vi "Main.vi"() -> ()   [LabVIEW 2021] (continued)
                    w821 = T9 37 items=["刷新间隔", "波特率", "布尔1设置项", "布尔2设置项", "布尔3设置项", "布尔4设置项", "布尔5设置项", "布尔6设置项", "布尔7设置项", "布尔8设置项", "显控1设置", "显控2设置", "显控3设置", "显控4设置", "显控5设置", "显控6设置", "显控7设置", "显控8设置", "显控9设置", "显控10设置", "显控11设置", "显控12设置", "设控1设置", "设控2设置", "设控3设置", "设控4设置", "设控5设置", "设控6设置", "设控7设置", "设控8设置", "曲线1设置", "曲线2设置", "曲线3设置", "曲线4设置", "曲线5设置", "曲线6设置", "曲线7设置", "曲线8设置", "曲线9设置", "曲线10设置", "曲线11设置", "曲线12设置", "曲线13设置", "曲线14设置", "曲线15设置", "曲线16设置", "曲线17设置", "曲线18设置", "曲线19设置", "曲线20设置", "曲线21设置", "曲线22设置", "曲线23设置", "曲线24设置", "曲线25设置", "曲线26设置", "曲线27设置", "曲线28设置", "曲线29设置", "曲线30设置", "曲线31设置", "曲线32设置", "曲线33设置", "曲线34设置", "曲线35设置", "曲线36设置", "曲线37设置", "曲线38设置", "曲线39设置", "曲线40设置", "曲线41设置", "曲线42设置", "曲线43设置", "曲线44设置", "曲线45设置", "曲线46设置", "曲线47设置", "曲线48设置", "曲线49设置", "曲线50设置", "曲线51设置", "曲线52设置", "曲线53设置", "曲线54设置", "曲线55设置", "曲线56设置", "曲线57设置", "曲线58设置", "曲线59设置", "曲线60设置", "曲线61设置", "曲线62设置", "曲线63设置", "曲线64设置", "ID值", "数据模式"] ("DataInitDef")
                    n650 = property on="表格" class="Tbl (严格)"() -> ("Selection Start"=w831:T1)  [unwired: 2 in, 2 out]
                    n651 = Unbundle By Name(w831) -> ("Row"=w829:i32)
                    n652 = property on="表格" class="Tbl (严格)"() -> ("Value"=w830:string[][])  [unwired: 2 in, 2 out]
                    n653 = Number To Decimal String(number=w829) -> (decimal integer string=w828:string)  [unwired: 1 in]
                    n654 = Index Array(array=w830, index (row)=w829, index (col)=0 ("禁用的索引 (列)")) -> (element=w827:string)
                    n655 = String Subset(string=w827, length (rest)=16 ("长度（剩余）")) -> (substring=w826:string)  [unwired: 1 in]
                    n656 = property on="曲线8设置" class="Str"("Val(Sgnl)"=w826) -> ()  [unwired: 2 in, 2 out]
                    n657 = invoke on="控件配置文件" class="Tbl (严格)" method="Set Cell Value"("X Index"=1 ("X索引"), "Y Index"=w821, "Value"=w828) -> ()  [unwired: 3 in, 6 out]
                    n658 = invoke on="控件配置文件" class="Tbl (严格)" method="Set Cell Value"("X Index"=0 ("X索引"), "Y Index"=w821, "Value"=w826) -> ()  [unwired: 3 in, 6 out]
                  }
                  frame "关联到曲线9" {
                    w832 = T9 38 items=["刷新间隔", "波特率", "布尔1设置项", "布尔2设置项", "布尔3设置项", "布尔4设置项", "布尔5设置项", "布尔6设置项", "布尔7设置项", "布尔8设置项", "显控1设置", "显控2设置", "显控3设置", "显控4设置", "显控5设置", "显控6设置", "显控7设置", "显控8设置", "显控9设置", "显控10设置", "显控11设置", "显控12设置", "设控1设置", "设控2设置", "设控3设置", "设控4设置", "设控5设置", "设控6设置", "设控7设置", "设控8设置", "曲线1设置", "曲线2设置", "曲线3设置", "曲线4设置", "曲线5设置", "曲线6设置", "曲线7设置", "曲线8设置", "曲线9设置", "曲线10设置", "曲线11设置", "曲线12设置", "曲线13设置", "曲线14设置", "曲线15设置", "曲线16设置", "曲线17设置", "曲线18设置", "曲线19设置", "曲线20设置", "曲线21设置", "曲线22设置", "曲线23设置", "曲线24设置", "曲线25设置", "曲线26设置", "曲线27设置", "曲线28设置", "曲线29设置", "曲线30设置", "曲线31设置", "曲线32设置", "曲线33设置", "曲线34设置", "曲线35设置", "曲线36设置", "曲线37设置", "曲线38设置", "曲线39设置", "曲线40设置", "曲线41设置", "曲线42设置", "曲线43设置", "曲线44设置", "曲线45设置", "曲线46设置", "曲线47设置", "曲线48设置", "曲线49设置", "曲线50设置", "曲线51设置", "曲线52设置", "曲线53设置", "曲线54设置", "曲线55设置", "曲线56设置", "曲线57设置", "曲线58设置", "曲线59设置", "曲线60设置", "曲线61设置", "曲线62设置", "曲线63设置", "曲线64设置", "ID值", "数据模式"] ("DataInitDef")
                    n659 = property on="表格" class="Tbl (严格)"() -> ("Selection Start"=w842:T1)  [unwired: 2 in, 2 out]
                    n660 = Unbundle By Name(w842) -> ("Row"=w840:i32)
                    n661 = property on="表格" class="Tbl (严格)"() -> ("Value"=w841:string[][])  [unwired: 2 in, 2 out]
                    n662 = Number To Decimal String(number=w840) -> (decimal integer string=w839:string)  [unwired: 1 in]
                    n663 = Index Array(array=w841, index (row)=w840, index (col)=0 ("禁用的索引 (列)")) -> (element=w838:string)
                    n664 = String Subset(string=w838, length (rest)=16 ("长度（剩余）")) -> (substring=w837:string)  [unwired: 1 in]
                    n665 = property on="曲线9设置" class="Str"("Val(Sgnl)"=w837) -> ()  [unwired: 2 in, 2 out]
                    n666 = invoke on="控件配置文件" class="Tbl (严格)" method="Set Cell Value"("X Index"=1 ("X索引"), "Y Index"=w832, "Value"=w839) -> ()  [unwired: 3 in, 6 out]
                    n667 = invoke on="控件配置文件" class="Tbl (严格)" method="Set Cell Value"("X Index"=0 ("X索引"), "Y Index"=w832, "Value"=w837) -> ()  [unwired: 3 in, 6 out]
                  }
                  frame "关联到曲线10" {
                    w843 = T9 39 items=["刷新间隔", "波特率", "布尔1设置项", "布尔2设置项", "布尔3设置项", "布尔4设置项", "布尔5设置项", "布尔6设置项", "布尔7设置项", "布尔8设置项", "显控1设置", "显控2设置", "显控3设置", "显控4设置", "显控5设置", "显控6设置", "显控7设置", "显控8设置", "显控9设置", "显控10设置", "显控11设置", "显控12设置", "设控1设置", "设控2设置", "设控3设置", "设控4设置", "设控5设置", "设控6设置", "设控7设置", "设控8设置", "曲线1设置", "曲线2设置", "曲线3设置", "曲线4设置", "曲线5设置", "曲线6设置", "曲线7设置", "曲线8设置", "曲线9设置", "曲线10设置", "曲线11设置", "曲线12设置", "曲线13设置", "曲线14设置", "曲线15设置", "曲线16设置", "曲线17设置", "曲线18设置", "曲线19设置", "曲线20设置", "曲线21设置", "曲线22设置", "曲线23设置", "曲线24设置", "曲线25设置", "曲线26设置", "曲线27设置", "曲线28设置", "曲线29设置", "曲线30设置", "曲线31设置", "曲线32设置", "曲线33设置", "曲线34设置", "曲线35设置", "曲线36设置", "曲线37设置", "曲线38设置", "曲线39设置", "曲线40设置", "曲线41设置", "曲线42设置", "曲线43设置", "曲线44设置", "曲线45设置", "曲线46设置", "曲线47设置", "曲线48设置", "曲线49设置", "曲线50设置", "曲线51设置", "曲线52设置", "曲线53设置", "曲线54设置", "曲线55设置", "曲线56设置", "曲线57设置", "曲线58设置", "曲线59设置", "曲线60设置", "曲线61设置", "曲线62设置", "曲线63设置", "曲线64设置", "ID值", "数据模式"] ("DataInitDef")
                    n668 = property on="表格" class="Tbl (严格)"() -> ("Selection Start"=w848:T1)  [unwired: 2 in, 2 out]
                    n669 = Unbundle By Name(w848) -> ("Row"=w850:i32)
                    n670 = property on="表格" class="Tbl (严格)"() -> ("Value"=w849:string[][])  [unwired: 2 in, 2 out]
                    n671 = Number To Decimal String(number=w850) -> (decimal integer string=w851:string)  [unwired: 1 in]
                    n672 = Index Array(array=w849, index (row)=w850, index (col)=0 ("禁用的索引 (列)")) -> (element=w852:string)
                    n673 = String Subset(string=w852, length (rest)=16 ("长度（剩余）")) -> (substring=w853:string)  [unwired: 1 in]
                    n674 = property on="曲线10设置" class="Str"("Val(Sgnl)"=w853) -> ()  [unwired: 2 in, 2 out]
                    n675 = invoke on="控件配置文件" class="Tbl (严格)" method="Set Cell Value"("X Index"=1 ("X索引"), "Y Index"=w843, "Value"=w851) -> ()  [unwired: 3 in, 6 out]
                    n676 = invoke on="控件配置文件" class="Tbl (严格)" method="Set Cell Value"("X Index"=0 ("X索引"), "Y Index"=w843, "Value"=w853) -> ()  [unwired: 3 in, 6 out]
                  }
                  frame "关联到曲线11" {
                    w854 = T9 40 items=["刷新间隔", "波特率", "布尔1设置项", "布尔2设置项", "布尔3设置项", "布尔4设置项", "布尔5设置项", "布尔6设置项", "布尔7设置项", "布尔8设置项", "显控1设置", "显控2设置", "显控3设置", "显控4设置", "显控5设置", "显控6设置", "显控7设置", "显控8设置", "显控9设置", "显控10设置", "显控11设置", "显控12设置", "设控1设置", "设控2设置", "设控3设置", "设控4设置", "设控5设置", "设控6设置", "设控7设置", "设控8设置", "曲线1设置", "曲线2设置", "曲线3设置", "曲线4设置", "曲线5设置", "曲线6设置", "曲线7设置", "曲线8设置", "曲线9设置", "曲线10设置", "曲线11设置", "曲线12设置", "曲线13设置", "曲线14设置", "曲线15设置", "曲线16设置", "曲线17设置", "曲线18设置", "曲线19设置", "曲线20设置", "曲线21设置", "曲线22设置", "曲线23设置", "曲线24设置", "曲线25设置", "曲线26设置", "曲线27设置", "曲线28设置", "曲线29设置", "曲线30设置", "曲线31设置", "曲线32设置", "曲线33设置", "曲线34设置", "曲线35设置", "曲线36设置", "曲线37设置", "曲线38设置", "曲线39设置", "曲线40设置", "曲线41设置", "曲线42设置", "曲线43设置", "曲线44设置", "曲线45设置", "曲线46设置", "曲线47设置", "曲线48设置", "曲线49设置", "曲线50设置", "曲线51设置", "曲线52设置", "曲线53设置", "曲线54设置", "曲线55设置", "曲线56设置", "曲线57设置", "曲线58设置", "曲线59设置", "曲线60设置", "曲线61设置", "曲线62设置", "曲线63设置", "曲线64设置", "ID值", "数据模式"] ("DataInitDef")
                    n677 = property on="表格" class="Tbl (严格)"() -> ("Selection Start"=w859:T1)  [unwired: 2 in, 2 out]
                    n678 = Unbundle By Name(w859) -> ("Row"=w861:i32)
                    n679 = property on="表格" class="Tbl (严格)"() -> ("Value"=w860:string[][])  [unwired: 2 in, 2 out]
                    n680 = Number To Decimal String(number=w861) -> (decimal integer string=w862:string)  [unwired: 1 in]
                    n681 = Index Array(array=w860, index (row)=w861, index (col)=0 ("禁用的索引 (列)")) -> (element=w863:string)
                    n682 = String Subset(string=w863, length (rest)=16 ("长度（剩余）")) -> (substring=w864:string)  [unwired: 1 in]
                    n683 = property on="曲线11设置" class="Str"("Val(Sgnl)"=w864) -> ()  [unwired: 2 in, 2 out]
                    n684 = invoke on="控件配置文件" class="Tbl (严格)" method="Set Cell Value"("X Index"=1 ("X索引"), "Y Index"=w854, "Value"=w862) -> ()  [unwired: 3 in, 6 out]
                    n685 = invoke on="控件配置文件" class="Tbl (严格)" method="Set Cell Value"("X Index"=0 ("X索引"), "Y Index"=w854, "Value"=w864) -> ()  [unwired: 3 in, 6 out]
                  }
                  frame "关联到曲线12" {
                    w865 = T9 41 items=["刷新间隔", "波特率", "布尔1设置项", "布尔2设置项", "布尔3设置项", "布尔4设置项", "布尔5设置项", "布尔6设置项", "布尔7设置项", "布尔8设置项", "显控1设置", "显控2设置", "显控3设置", "显控4设置", "显控5设置", "显控6设置", "显控7设置", "显控8设置", "显控9设置", "显控10设置", "显控11设置", "显控12设置", "设控1设置", "设控2设置", "设控3设置", "设控4设置", "设控5设置", "设控6设置", "设控7设置", "设控8设置", "曲线1设置", "曲线2设置", "曲线3设置", "曲线4设置", "曲线5设置", "曲线6设置", "曲线7设置", "曲线8设置", "曲线9设置", "曲线10设置", "曲线11设置", "曲线12设置", "曲线13设置", "曲线14设置", "曲线15设置", "曲线16设置", "曲线17设置", "曲线18设置", "曲线19设置", "曲线20设置", "曲线21设置", "曲线22设置", "曲线23设置", "曲线24设置", "曲线25设置", "曲线26设置", "曲线27设置", "曲线28设置", "曲线29设置", "曲线30设置", "曲线31设置", "曲线32设置", "曲线33设置", "曲线34设置", "曲线35设置", "曲线36设置", "曲线37设置", "曲线38设置", "曲线39设置", "曲线40设置", "曲线41设置", "曲线42设置", "曲线43设置", "曲线44设置", "曲线45设置", "曲线46设置", "曲线47设置", "曲线48设置", "曲线49设置", "曲线50设置", "曲线51设置", "曲线52设置", "曲线53设置", "曲线54设置", "曲线55设置", "曲线56设置", "曲线57设置", "曲线58设置", "曲线59设置", "曲线60设置", "曲线61设置", "曲线62设置", "曲线63设置", "曲线64设置", "ID值", "数据模式"] ("DataInitDef")
                    n686 = property on="表格" class="Tbl (严格)"() -> ("Selection Start"=w870:T1)  [unwired: 2 in, 2 out]
                    n687 = Unbundle By Name(w870) -> ("Row"=w872:i32)
                    n688 = property on="表格" class="Tbl (严格)"() -> ("Value"=w871:string[][])  [unwired: 2 in, 2 out]
                    n689 = Number To Decimal String(number=w872) -> (decimal integer string=w873:string)  [unwired: 1 in]
                    n690 = Index Array(array=w871, index (row)=w872, index (col)=0 ("禁用的索引 (列)")) -> (element=w874:string)
                    n691 = String Subset(string=w874, length (rest)=16 ("长度（剩余）")) -> (substring=w875:string)  [unwired: 1 in]
                    n692 = property on="曲线12设置" class="Str"("Val(Sgnl)"=w875) -> ()  [unwired: 2 in, 2 out]
                    n693 = invoke on="控件配置文件" class="Tbl (严格)" method="Set Cell Value"("X Index"=1 ("X索引"), "Y Index"=w865, "Value"=w873) -> ()  [unwired: 3 in, 6 out]
                    n694 = invoke on="控件配置文件" class="Tbl (严格)" method="Set Cell Value"("X Index"=0 ("X索引"), "Y Index"=w865, "Value"=w875) -> ()  [unwired: 3 in, 6 out]
                  }
                  frame "关联到曲线13" {
                    w876 = T9 42 items=["刷新间隔", "波特率", "布尔1设置项", "布尔2设置项", "布尔3设置项", "布尔4设置项", "布尔5设置项", "布尔6设置项", "布尔7设置项", "布尔8设置项", "显控1设置", "显控2设置", "显控3设置", "显控4设置", "显控5设置", "显控6设置", "显控7设置", "显控8设置", "显控9设置", "显控10设置", "显控11设置", "显控12设置", "设控1设置", "设控2设置", "设控3设置", "设控4设置", "设控5设置", "设控6设置", "设控7设置", "设控8设置", "曲线1设置", "曲线2设置", "曲线3设置", "曲线4设置", "曲线5设置", "曲线6设置", "曲线7设置", "曲线8设置", "曲线9设置", "曲线10设置", "曲线11设置", "曲线12设置", "曲线13设置", "曲线14设置", "曲线15设置", "曲线16设置", "曲线17设置", "曲线18设置", "曲线19设置", "曲线20设置", "曲线21设置", "曲线22设置", "曲线23设置", "曲线24设置", "曲线25设置", "曲线26设置", "曲线27设置", "曲线28设置", "曲线29设置", "曲线30设置", "曲线31设置", "曲线32设置", "曲线33设置", "曲线34设置", "曲线35设置", "曲线36设置", "曲线37设置", "曲线38设置", "曲线39设置", "曲线40设置", "曲线41设置", "曲线42设置", "曲线43设置", "曲线44设置", "曲线45设置", "曲线46设置", "曲线47设置", "曲线48设置", "曲线49设置", "曲线50设置", "曲线51设置", "曲线52设置", "曲线53设置", "曲线54设置", "曲线55设置", "曲线56设置", "曲线57设置", "曲线58设置", "曲线59设置", "曲线60设置", "曲线61设置", "曲线62设置", "曲线63设置", "曲线64设置", "ID值", "数据模式"] ("DataInitDef")
                    n695 = property on="表格" class="Tbl (严格)"() -> ("Selection Start"=w881:T1)  [unwired: 2 in, 2 out]
                    n696 = Unbundle By Name(w881) -> ("Row"=w883:i32)
                    n697 = property on="表格" class="Tbl (严格)"() -> ("Value"=w882:string[][])  [unwired: 2 in, 2 out]
                    n698 = Number To Decimal String(number=w883) -> (decimal integer string=w884:string)  [unwired: 1 in]
                    n699 = Index Array(array=w882, index (row)=w883, index (col)=0 ("禁用的索引 (列)")) -> (element=w885:string)
                    n700 = String Subset(string=w885, length (rest)=16 ("长度（剩余）")) -> (substring=w886:string)  [unwired: 1 in]
                    n701 = property on="曲线13设置" class="Str"("Val(Sgnl)"=w886) -> ()  [unwired: 2 in, 2 out]
                    n702 = invoke on="控件配置文件" class="Tbl (严格)" method="Set Cell Value"("X Index"=1 ("X索引"), "Y Index"=w876, "Value"=w884) -> ()  [unwired: 3 in, 6 out]
                    n703 = invoke on="控件配置文件" class="Tbl (严格)" method="Set Cell Value"("X Index"=0 ("X索引"), "Y Index"=w876, "Value"=w886) -> ()  [unwired: 3 in, 6 out]
                  }
                  frame "关联到曲线14" {
                    w887 = T9 43 items=["刷新间隔", "波特率", "布尔1设置项", "布尔2设置项", "布尔3设置项", "布尔4设置项", "布尔5设置项", "布尔6设置项", "布尔7设置项", "布尔8设置项", "显控1设置", "显控2设置", "显控3设置", "显控4设置", "显控5设置", "显控6设置", "显控7设置", "显控8设置", "显控9设置", "显控10设置", "显控11设置", "显控12设置", "设控1设置", "设控2设置", "设控3设置", "设控4设置", "设控5设置", "设控6设置", "设控7设置", "设控8设置", "曲线1设置", "曲线2设置", "曲线3设置", "曲线4设置", "曲线5设置", "曲线6设置", "曲线7设置", "曲线8设置", "曲线9设置", "曲线10设置", "曲线11设置", "曲线12设置", "曲线13设置", "曲线14设置", "曲线15设置", "曲线16设置", "曲线17设置", "曲线18设置", "曲线19设置", "曲线20设置", "曲线21设置", "曲线22设置", "曲线23设置", "曲线24设置", "曲线25设置", "曲线26设置", "曲线27设置", "曲线28设置", "曲线29设置", "曲线30设置", "曲线31设置", "曲线32设置", "曲线33设置", "曲线34设置", "曲线35设置", "曲线36设置", "曲线37设置", "曲线38设置", "曲线39设置", "曲线40设置", "曲线41设置", "曲线42设置", "曲线43设置", "曲线44设置", "曲线45设置", "曲线46设置", "曲线47设置", "曲线48设置", "曲线49设置", "曲线50设置", "曲线51设置", "曲线52设置", "曲线53设置", "曲线54设置", "曲线55设置", "曲线56设置", "曲线57设置", "曲线58设置", "曲线59设置", "曲线60设置", "曲线61设置", "曲线62设置", "曲线63设置", "曲线64设置", "ID值", "数据模式"] ("DataInitDef")
                    n704 = property on="表格" class="Tbl (严格)"() -> ("Selection Start"=w892:T1)  [unwired: 2 in, 2 out]
                    n705 = Unbundle By Name(w892) -> ("Row"=w894:i32)
                    n706 = property on="表格" class="Tbl (严格)"() -> ("Value"=w893:string[][])  [unwired: 2 in, 2 out]
                    n707 = Number To Decimal String(number=w894) -> (decimal integer string=w895:string)  [unwired: 1 in]
                    n708 = Index Array(array=w893, index (row)=w894, index (col)=0 ("禁用的索引 (列)")) -> (element=w896:string)
                    n709 = String Subset(string=w896, length (rest)=16 ("长度（剩余）")) -> (substring=w897:string)  [unwired: 1 in]
                    n710 = property on="曲线14设置" class="Str"("Val(Sgnl)"=w897) -> ()  [unwired: 2 in, 2 out]
                    n711 = invoke on="控件配置文件" class="Tbl (严格)" method="Set Cell Value"("X Index"=1 ("X索引"), "Y Index"=w887, "Value"=w895) -> ()  [unwired: 3 in, 6 out]
                    n712 = invoke on="控件配置文件" class="Tbl (严格)" method="Set Cell Value"("X Index"=0 ("X索引"), "Y Index"=w887, "Value"=w897) -> ()  [unwired: 3 in, 6 out]
                  }
                  frame "关联到曲线15" {
                    w898 = T9 44 items=["刷新间隔", "波特率", "布尔1设置项", "布尔2设置项", "布尔3设置项", "布尔4设置项", "布尔5设置项", "布尔6设置项", "布尔7设置项", "布尔8设置项", "显控1设置", "显控2设置", "显控3设置", "显控4设置", "显控5设置", "显控6设置", "显控7设置", "显控8设置", "显控9设置", "显控10设置", "显控11设置", "显控12设置", "设控1设置", "设控2设置", "设控3设置", "设控4设置", "设控5设置", "设控6设置", "设控7设置", "设控8设置", "曲线1设置", "曲线2设置", "曲线3设置", "曲线4设置", "曲线5设置", "曲线6设置", "曲线7设置", "曲线8设置", "曲线9设置", "曲线10设置", "曲线11设置", "曲线12设置", "曲线13设置", "曲线14设置", "曲线15设置", "曲线16设置", "曲线17设置", "曲线18设置", "曲线19设置", "曲线20设置", "曲线21设置", "曲线22设置", "曲线23设置", "曲线24设置", "曲线25设置", "曲线26设置", "曲线27设置", "曲线28设置", "曲线29设置", "曲线30设置", "曲线31设置", "曲线32设置", "曲线33设置", "曲线34设置", "曲线35设置", "曲线36设置", "曲线37设置", "曲线38设置", "曲线39设置", "曲线40设置", "曲线41设置", "曲线42设置", "曲线43设置", "曲线44设置", "曲线45设置", "曲线46设置", "曲线47设置", "曲线48设置", "曲线49设置", "曲线50设置", "曲线51设置", "曲线52设置", "曲线53设置", "曲线54设置", "曲线55设置", "曲线56设置", "曲线57设置", "曲线58设置", "曲线59设置", "曲线60设置", "曲线61设置", "曲线62设置", "曲线63设置", "曲线64设置", "ID值", "数据模式"] ("DataInitDef")
                    n713 = property on="表格" class="Tbl (严格)"() -> ("Selection Start"=w903:T1)  [unwired: 2 in, 2 out]
                    n714 = Unbundle By Name(w903) -> ("Row"=w905:i32)
                    n715 = property on="表格" class="Tbl (严格)"() -> ("Value"=w904:string[][])  [unwired: 2 in, 2 out]
                    n716 = Number To Decimal String(number=w905) -> (decimal integer string=w906:string)  [unwired: 1 in]
                    n717 = Index Array(array=w904, index (row)=w905, index (col)=0 ("禁用的索引 (列)")) -> (element=w907:string)
                    n718 = String Subset(string=w907, length (rest)=16 ("长度（剩余）")) -> (substring=w908:string)  [unwired: 1 in]
                    n719 = property on="曲线15设置" class="Str"("Val(Sgnl)"=w908) -> ()  [unwired: 2 in, 2 out]
                    n720 = invoke on="控件配置文件" class="Tbl (严格)" method="Set Cell Value"("X Index"=1 ("X索引"), "Y Index"=w898, "Value"=w906) -> ()  [unwired: 3 in, 6 out]
                    n721 = invoke on="控件配置文件" class="Tbl (严格)" method="Set Cell Value"("X Index"=0 ("X索引"), "Y Index"=w898, "Value"=w908) -> ()  [unwired: 3 in, 6 out]
                  }
                  frame "关联到曲线16" {
                    w909 = T9 45 items=["刷新间隔", "波特率", "布尔1设置项", "布尔2设置项", "布尔3设置项", "布尔4设置项", "布尔5设置项", "布尔6设置项", "布尔7设置项", "布尔8设置项", "显控1设置", "显控2设置", "显控3设置", "显控4设置", "显控5设置", "显控6设置", "显控7设置", "显控8设置", "显控9设置", "显控10设置", "显控11设置", "显控12设置", "设控1设置", "设控2设置", "设控3设置", "设控4设置", "设控5设置", "设控6设置", "设控7设置", "设控8设置", "曲线1设置", "曲线2设置", "曲线3设置", "曲线4设置", "曲线5设置", "曲线6设置", "曲线7设置", "曲线8设置", "曲线9设置", "曲线10设置", "曲线11设置", "曲线12设置", "曲线13设置", "曲线14设置", "曲线15设置", "曲线16设置", "曲线17设置", "曲线18设置", "曲线19设置", "曲线20设置", "曲线21设置", "曲线22设置", "曲线23设置", "曲线24设置", "曲线25设置", "曲线26设置", "曲线27设置", "曲线28设置", "曲线29设置", "曲线30设置", "曲线31设置", "曲线32设置", "曲线33设置", "曲线34设置", "曲线35设置", "曲线36设置", "曲线37设置", "曲线38设置", "曲线39设置", "曲线40设置", "曲线41设置", "曲线42设置", "曲线43设置", "曲线44设置", "曲线45设置", "曲线46设置", "曲线47设置", "曲线48设置", "曲线49设置", "曲线50设置", "曲线51设置", "曲线52设置", "曲线53设置", "曲线54设置", "曲线55设置", "曲线56设置", "曲线57设置", "曲线58设置", "曲线59设置", "曲线60设置", "曲线61设置", "曲线62设置", "曲线63设置", "曲线64设置", "ID值", "数据模式"] ("DataInitDef")
                    n722 = property on="表格" class="Tbl (严格)"() -> ("Selection Start"=w919:T1)  [unwired: 2 in, 2 out]
                    n723 = Unbundle By Name(w919) -> ("Row"=w917:i32)
                    n724 = property on="表格" class="Tbl (严格)"() -> ("Value"=w918:string[][])  [unwired: 2 in, 2 out]
                    n725 = Number To Decimal String(number=w917) -> (decimal integer string=w916:string)  [unwired: 1 in]
                    n726 = Index Array(array=w918, index (row)=w917, index (col)=0 ("禁用的索引 (列)")) -> (element=w915:string)
                    n727 = String Subset(string=w915, length (rest)=16 ("长度（剩余）")) -> (substring=w914:string)  [unwired: 1 in]
                    n728 = property on="曲线16设置" class="Str"("Val(Sgnl)"=w914) -> ()  [unwired: 2 in, 2 out]
                    n729 = invoke on="控件配置文件" class="Tbl (严格)" method="Set Cell Value"("X Index"=1 ("X索引"), "Y Index"=w909, "Value"=w916) -> ()  [unwired: 3 in, 6 out]
                    n730 = invoke on="控件配置文件" class="Tbl (严格)" method="Set Cell Value"("X Index"=0 ("X索引"), "Y Index"=w909, "Value"=w914) -> ()  [unwired: 3 in, 6 out]
                  }
                  frame "关联到曲线17" {
                    w920 = T9 46 items=["刷新间隔", "波特率", "布尔1设置项", "布尔2设置项", "布尔3设置项", "布尔4设置项", "布尔5设置项", "布尔6设置项", "布尔7设置项", "布尔8设置项", "显控1设置", "显控2设置", "显控3设置", "显控4设置", "显控5设置", "显控6设置", "显控7设置", "显控8设置", "显控9设置", "显控10设置", "显控11设置", "显控12设置", "设控1设置", "设控2设置", "设控3设置", "设控4设置", "设控5设置", "设控6设置", "设控7设置", "设控8设置", "曲线1设置", "曲线2设置", "曲线3设置", "曲线4设置", "曲线5设置", "曲线6设置", "曲线7设置", "曲线8设置", "曲线9设置", "曲线10设置", "曲线11设置", "曲线12设置", "曲线13设置", "曲线14设置", "曲线15设置", "曲线16设置", "曲线17设置", "曲线18设置", "曲线19设置", "曲线20设置", "曲线21设置", "曲线22设置", "曲线23设置", "曲线24设置", "曲线25设置", "曲线26设置", "曲线27设置", "曲线28设置", "曲线29设置", "曲线30设置", "曲线31设置", "曲线32设置", "曲线33设置", "曲线34设置", "曲线35设置", "曲线36设置", "曲线37设置", "曲线38设置", "曲线39设置", "曲线40设置", "曲线41设置", "曲线42设置", "曲线43设置", "曲线44设置", "曲线45设置", "曲线46设置", "曲线47设置", "曲线48设置", "曲线49设置", "曲线50设置", "曲线51设置", "曲线52设置", "曲线53设置", "曲线54设置", "曲线55设置", "曲线56设置", "曲线57设置", "曲线58设置", "曲线59设置", "曲线60设置", "曲线61设置", "曲线62设置", "曲线63设置", "曲线64设置", "ID值", "数据模式"] ("DataInitDef")
                    n731 = property on="表格" class="Tbl (严格)"() -> ("Selection Start"=w930:T1)  [unwired: 2 in, 2 out]
                    n732 = Unbundle By Name(w930) -> ("Row"=w928:i32)
                    n733 = property on="表格" class="Tbl (严格)"() -> ("Value"=w929:string[][])  [unwired: 2 in, 2 out]
                    n734 = Number To Decimal String(number=w928) -> (decimal integer string=w927:string)  [unwired: 1 in]
                    n735 = Index Array(array=w929, index (row)=w928, index (col)=0 ("禁用的索引 (列)")) -> (element=w926:string)
                    n736 = String Subset(string=w926, length (rest)=16 ("长度（剩余）")) -> (substring=w925:string)  [unwired: 1 in]
                    n737 = property on="曲线17设置" class="Str"("Val(Sgnl)"=w925) -> ()  [unwired: 2 in, 2 out]
                    n738 = invoke on="控件配置文件" class="Tbl (严格)" method="Set Cell Value"("X Index"=1 ("X索引"), "Y Index"=w920, "Value"=w927) -> ()  [unwired: 3 in, 6 out]
                    n739 = invoke on="控件配置文件" class="Tbl (严格)" method="Set Cell Value"("X Index"=0 ("X索引"), "Y Index"=w920, "Value"=w925) -> ()  [unwired: 3 in, 6 out]
                  }
                  frame "关联到曲线18" {
                    w931 = T9 47 items=["刷新间隔", "波特率", "布尔1设置项", "布尔2设置项", "布尔3设置项", "布尔4设置项", "布尔5设置项", "布尔6设置项", "布尔7设置项", "布尔8设置项", "显控1设置", "显控2设置", "显控3设置", "显控4设置", "显控5设置", "显控6设置", "显控7设置", "显控8设置", "显控9设置", "显控10设置", "显控11设置", "显控12设置", "设控1设置", "设控2设置", "设控3设置", "设控4设置", "设控5设置", "设控6设置", "设控7设置", "设控8设置", "曲线1设置", "曲线2设置", "曲线3设置", "曲线4设置", "曲线5设置", "曲线6设置", "曲线7设置", "曲线8设置", "曲线9设置", "曲线10设置", "曲线11设置", "曲线12设置", "曲线13设置", "曲线14设置", "曲线15设置", "曲线16设置", "曲线17设置", "曲线18设置", "曲线19设置", "曲线20设置", "曲线21设置", "曲线22设置", "曲线23设置", "曲线24设置", "曲线25设置", "曲线26设置", "曲线27设置", "曲线28设置", "曲线29设置", "曲线30设置", "曲线31设置", "曲线32设置", "曲线33设置", "曲线34设置", "曲线35设置", "曲线36设置", "曲线37设置", "曲线38设置", "曲线39设置", "曲线40设置", "曲线41设置", "曲线42设置", "曲线43设置", "曲线44设置", "曲线45设置", "曲线46设置", "曲线47设置", "曲线48设置", "曲线49设置", "曲线50设置", "曲线51设置", "曲线52设置", "曲线53设置", "曲线54设置", "曲线55设置", "曲线56设置", "曲线57设置", "曲线58设置", "曲线59设置", "曲线60设置", "曲线61设置", "曲线62设置", "曲线63设置", "曲线64设置", "ID值", "数据模式"] ("DataInitDef")
                    n740 = property on="表格" class="Tbl (严格)"() -> ("Selection Start"=w941:T1)  [unwired: 2 in, 2 out]
                    n741 = Unbundle By Name(w941) -> ("Row"=w939:i32)
                    n742 = property on="表格" class="Tbl (严格)"() -> ("Value"=w940:string[][])  [unwired: 2 in, 2 out]
                    n743 = Number To Decimal String(number=w939) -> (decimal integer string=w938:string)  [unwired: 1 in]
                    n744 = Index Array(array=w940, index (row)=w939, index (col)=0 ("禁用的索引 (列)")) -> (element=w937:string)
                    n745 = String Subset(string=w937, length (rest)=16 ("长度（剩余）")) -> (substring=w936:string)  [unwired: 1 in]
                    n746 = property on="曲线18设置" class="Str"("Val(Sgnl)"=w936) -> ()  [unwired: 2 in, 2 out]
                    n747 = invoke on="控件配置文件" class="Tbl (严格)" method="Set Cell Value"("X Index"=1 ("X索引"), "Y Index"=w931, "Value"=w938) -> ()  [unwired: 3 in, 6 out]
                    n748 = invoke on="控件配置文件" class="Tbl (严格)" method="Set Cell Value"("X Index"=0 ("X索引"), "Y Index"=w931, "Value"=w936) -> ()  [unwired: 3 in, 6 out]
                  }
                  frame "关联到曲线19" {
                    w942 = T9 48 items=["刷新间隔", "波特率", "布尔1设置项", "布尔2设置项", "布尔3设置项", "布尔4设置项", "布尔5设置项", "布尔6设置项", "布尔7设置项", "布尔8设置项", "显控1设置", "显控2设置", "显控3设置", "显控4设置", "显控5设置", "显控6设置", "显控7设置", "显控8设置", "显控9设置", "显控10设置", "显控11设置", "显控12设置", "设控1设置", "设控2设置", "设控3设置", "设控4设置", "设控5设置", "设控6设置", "设控7设置", "设控8设置", "曲线1设置", "曲线2设置", "曲线3设置", "曲线4设置", "曲线5设置", "曲线6设置", "曲线7设置", "曲线8设置", "曲线9设置", "曲线10设置", "曲线11设置", "曲线12设置", "曲线13设置", "曲线14设置", "曲线15设置", "曲线16设置", "曲线17设置", "曲线18设置", "曲线19设置", "曲线20设置", "曲线21设置", "曲线22设置", "曲线23设置", "曲线24设置", "曲线25设置", "曲线26设置", "曲线27设置", "曲线28设置", "曲线29设置", "曲线30设置", "曲线31设置", "曲线32设置", "曲线33设置", "曲线34设置", "曲线35设置", "曲线36设置", "曲线37设置", "曲线38设置", "曲线39设置", "曲线40设置", "曲线41设置", "曲线42设置", "曲线43设置", "曲线44设置", "曲线45设置", "曲线46设置", "曲线47设置", "曲线48设置", "曲线49设置", "曲线50设置", "曲线51设置", "曲线52设置", "曲线53设置", "曲线54设置", "曲线55设置", "曲线56设置", "曲线57设置", "曲线58设置", "曲线59设置", "曲线60设置", "曲线61设置", "曲线62设置", "曲线63设置", "曲线64设置", "ID值", "数据模式"] ("DataInitDef")
                    n749 = property on="表格" class="Tbl (严格)"() -> ("Selection Start"=w952:T1)  [unwired: 2 in, 2 out]
                    n750 = Unbundle By Name(w952) -> ("Row"=w950:i32)
                    n751 = property on="表格" class="Tbl (严格)"() -> ("Value"=w951:string[][])  [unwired: 2 in, 2 out]
                    n752 = Number To Decimal String(number=w950) -> (decimal integer string=w949:string)  [unwired: 1 in]
                    n753 = Index Array(array=w951, index (row)=w950, index (col)=0 ("禁用的索引 (列)")) -> (element=w948:string)
                    n754 = String Subset(string=w948, length (rest)=16 ("长度（剩余）")) -> (substring=w947:string)  [unwired: 1 in]
                    n755 = property on="曲线19设置" class="Str"("Val(Sgnl)"=w947) -> ()  [unwired: 2 in, 2 out]
                    n756 = invoke on="控件配置文件" class="Tbl (严格)" method="Set Cell Value"("X Index"=1 ("X索引"), "Y Index"=w942, "Value"=w949) -> ()  [unwired: 3 in, 6 out]
                    n757 = invoke on="控件配置文件" class="Tbl (严格)" method="Set Cell Value"("X Index"=0 ("X索引"), "Y Index"=w942, "Value"=w947) -> ()  [unwired: 3 in, 6 out]
                  }
                  frame "关联到曲线20" {
                    w953 = T9 49 items=["刷新间隔", "波特率", "布尔1设置项", "布尔2设置项", "布尔3设置项", "布尔4设置项", "布尔5设置项", "布尔6设置项", "布尔7设置项", "布尔8设置项", "显控1设置", "显控2设置", "显控3设置", "显控4设置", "显控5设置", "显控6设置", "显控7设置", "显控8设置", "显控9设置", "显控10设置", "显控11设置", "显控12设置", "设控1设置", "设控2设置", "设控3设置", "设控4设置", "设控5设置", "设控6设置", "设控7设置", "设控8设置", "曲线1设置", "曲线2设置", "曲线3设置", "曲线4设置", "曲线5设置", "曲线6设置", "曲线7设置", "曲线8设置", "曲线9设置", "曲线10设置", "曲线11设置", "曲线12设置", "曲线13设置", "曲线14设置", "曲线15设置", "曲线16设置", "曲线17设置", "曲线18设置", "曲线19设置", "曲线20设置", "曲线21设置", "曲线22设置", "曲线23设置", "曲线24设置", "曲线25设置", "曲线26设置", "曲线27设置", "曲线28设置", "曲线29设置", "曲线30设置", "曲线31设置", "曲线32设置", "曲线33设置", "曲线34设置", "曲线35设置", "曲线36设置", "曲线37设置", "曲线38设置", "曲线39设置", "曲线40设置", "曲线41设置", "曲线42设置", "曲线43设置", "曲线44设置", "曲线45设置", "曲线46设置", "曲线47设置", "曲线48设置", "曲线49设置", "曲线50设置", "曲线51设置", "曲线52设置", "曲线53设置", "曲线54设置", "曲线55设置", "曲线56设置", "曲线57设置", "曲线58设置", "曲线59设置", "曲线60设置", "曲线61设置", "曲线62设置", "曲线63设置", "曲线64设置", "ID值", "数据模式"] ("DataInitDef")
                    n758 = property on="表格" class="Tbl (严格)"() -> ("Selection Start"=w963:T1)  [unwired: 2 in, 2 out]
                    n759 = Unbundle By Name(w963) -> ("Row"=w961:i32)
                    n760 = property on="表格" class="Tbl (严格)"() -> ("Value"=w962:string[][])  [unwired: 2 in, 2 out]
                    n761 = Number To Decimal String(number=w961) -> (decimal integer string=w960:string)  [unwired: 1 in]
                    n762 = Index Array(array=w962, index (row)=w961, index (col)=0 ("禁用的索引 (列)")) -> (element=w959:string)
                    n763 = String Subset(string=w959, length (rest)=16 ("长度（剩余）")) -> (substring=w958:string)  [unwired: 1 in]
                    n764 = property on="曲线20设置" class="Str"("Val(Sgnl)"=w958) -> ()  [unwired: 2 in, 2 out]
                    n765 = invoke on="控件配置文件" class="Tbl (严格)" method="Set Cell Value"("X Index"=1 ("X索引"), "Y Index"=w953, "Value"=w960) -> ()  [unwired: 3 in, 6 out]
                    n766 = invoke on="控件配置文件" class="Tbl (严格)" method="Set Cell Value"("X Index"=0 ("X索引"), "Y Index"=w953, "Value"=w958) -> ()  [unwired: 3 in, 6 out]
                  }
                  frame "关联到曲线21" {
                    w964 = T9 50 items=["刷新间隔", "波特率", "布尔1设置项", "布尔2设置项", "布尔3设置项", "布尔4设置项", "布尔5设置项", "布尔6设置项", "布尔7设置项", "布尔8设置项", "显控1设置", "显控2设置", "显控3设置", "显控4设置", "显控5设置", "显控6设置", "显控7设置", "显控8设置", "显控9设置", "显控10设置", "显控11设置", "显控12设置", "设控1设置", "设控2设置", "设控3设置", "设控4设置", "设控5设置", "设控6设置", "设控7设置", "设控8设置", "曲线1设置", "曲线2设置", "曲线3设置", "曲线4设置", "曲线5设置", "曲线6设置", "曲线7设置", "曲线8设置", "曲线9设置", "曲线10设置", "曲线11设置", "曲线12设置", "曲线13设置", "曲线14设置", "曲线15设置", "曲线16设置", "曲线17设置", "曲线18设置", "曲线19设置", "曲线20设置", "曲线21设置", "曲线22设置", "曲线23设置", "曲线24设置", "曲线25设置", "曲线26设置", "曲线27设置", "曲线28设置", "曲线29设置", "曲线30设置", "曲线31设置", "曲线32设置", "曲线33设置", "曲线34设置", "曲线35设置", "曲线36设置", "曲线37设置", "曲线38设置", "曲线39设置", "曲线40设置", "曲线41设置", "曲线42设置", "曲线43设置", "曲线44设置", "曲线45设置", "曲线46设置", "曲线47设置", "曲线48设置", "曲线49设置", "曲线50设置", "曲线51设置", "曲线52设置", "曲线53设置", "曲线54设置", "曲线55设置", "曲线56设置", "曲线57设置", "曲线58设置", "曲线59设置", "曲线60设置", "曲线61设置", "曲线62设置", "曲线63设置", "曲线64设置", "ID值", "数据模式"] ("DataInitDef")
                    n767 = property on="表格" class="Tbl (严格)"() -> ("Selection Start"=w974:T1)  [unwired: 2 in, 2 out]
                    n768 = Unbundle By Name(w974) -> ("Row"=w972:i32)
                    n769 = property on="表格" class="Tbl (严格)"() -> ("Value"=w973:string[][])  [unwired: 2 in, 2 out]
                    n770 = Number To Decimal String(number=w972) -> (decimal integer string=w971:string)  [unwired: 1 in]
                    n771 = Index Array(array=w973, index (row)=w972, index (col)=0 ("禁用的索引 (列)")) -> (element=w970:string)
                    n772 = String Subset(string=w970, length (rest)=16 ("长度（剩余）")) -> (substring=w969:string)  [unwired: 1 in]
                    n773 = property on="曲线21设置" class="Str"("Val(Sgnl)"=w969) -> ()  [unwired: 2 in, 2 out]
                    n774 = invoke on="控件配置文件" class="Tbl (严格)" method="Set Cell Value"("X Index"=1 ("X索引"), "Y Index"=w964, "Value"=w971) -> ()  [unwired: 3 in, 6 out]
                    n775 = invoke on="控件配置文件" class="Tbl (严格)" method="Set Cell Value"("X Index"=0 ("X索引"), "Y Index"=w964, "Value"=w969) -> ()  [unwired: 3 in, 6 out]
                  }
                  frame "关联到曲线22" {
                    w975 = T9 51 items=["刷新间隔", "波特率", "布尔1设置项", "布尔2设置项", "布尔3设置项", "布尔4设置项", "布尔5设置项", "布尔6设置项", "布尔7设置项", "布尔8设置项", "显控1设置", "显控2设置", "显控3设置", "显控4设置", "显控5设置", "显控6设置", "显控7设置", "显控8设置", "显控9设置", "显控10设置", "显控11设置", "显控12设置", "设控1设置", "设控2设置", "设控3设置", "设控4设置", "设控5设置", "设控6设置", "设控7设置", "设控8设置", "曲线1设置", "曲线2设置", "曲线3设置", "曲线4设置", "曲线5设置", "曲线6设置", "曲线7设置", "曲线8设置", "曲线9设置", "曲线10设置", "曲线11设置", "曲线12设置", "曲线13设置", "曲线14设置", "曲线15设置", "曲线16设置", "曲线17设置", "曲线18设置", "曲线19设置", "曲线20设置", "曲线21设置", "曲线22设置", "曲线23设置", "曲线24设置", "曲线25设置", "曲线26设置", "曲线27设置", "曲线28设置", "曲线29设置", "曲线30设置", "曲线31设置", "曲线32设置", "曲线33设置", "曲线34设置", "曲线35设置", "曲线36设置", "曲线37设置", "曲线38设置", "曲线39设置", "曲线40设置", "曲线41设置", "曲线42设置", "曲线43设置", "曲线44设置", "曲线45设置", "曲线46设置", "曲线47设置", "曲线48设置", "曲线49设置", "曲线50设置", "曲线51设置", "曲线52设置", "曲线53设置", "曲线54设置", "曲线55设置", "曲线56设置", "曲线57设置", "曲线58设置", "曲线59设置", "曲线60设置", "曲线61设置", "曲线62设置", "曲线63设置", "曲线64设置", "ID值", "数据模式"] ("DataInitDef")
                    n776 = property on="表格" class="Tbl (严格)"() -> ("Selection Start"=w985:T1)  [unwired: 2 in, 2 out]
                    n777 = Unbundle By Name(w985) -> ("Row"=w983:i32)
                    n778 = property on="表格" class="Tbl (严格)"() -> ("Value"=w984:string[][])  [unwired: 2 in, 2 out]
                    n779 = Number To Decimal String(number=w983) -> (decimal integer string=w982:string)  [unwired: 1 in]
                    n780 = Index Array(array=w984, index (row)=w983, index (col)=0 ("禁用的索引 (列)")) -> (element=w981:string)
                    n781 = String Subset(string=w981, length (rest)=16 ("长度（剩余）")) -> (substring=w980:string)  [unwired: 1 in]
                    n782 = property on="曲线22设置" class="Str"("Val(Sgnl)"=w980) -> ()  [unwired: 2 in, 2 out]
                    n783 = invoke on="控件配置文件" class="Tbl (严格)" method="Set Cell Value"("X Index"=1 ("X索引"), "Y Index"=w975, "Value"=w982) -> ()  [unwired: 3 in, 6 out]
                    n784 = invoke on="控件配置文件" class="Tbl (严格)" method="Set Cell Value"("X Index"=0 ("X索引"), "Y Index"=w975, "Value"=w980) -> ()  [unwired: 3 in, 6 out]
                  }
                  frame "关联到曲线23" {
                    w986 = T9 52 items=["刷新间隔", "波特率", "布尔1设置项", "布尔2设置项", "布尔3设置项", "布尔4设置项", "布尔5设置项", "布尔6设置项", "布尔7设置项", "布尔8设置项", "显控1设置", "显控2设置", "显控3设置", "显控4设置", "显控5设置", "显控6设置", "显控7设置", "显控8设置", "显控9设置", "显控10设置", "显控11设置", "显控12设置", "设控1设置", "设控2设置", "设控3设置", "设控4设置", "设控5设置", "设控6设置", "设控7设置", "设控8设置", "曲线1设置", "曲线2设置", "曲线3设置", "曲线4设置", "曲线5设置", "曲线6设置", "曲线7设置", "曲线8设置", "曲线9设置", "曲线10设置", "曲线11设置", "曲线12设置", "曲线13设置", "曲线14设置", "曲线15设置", "曲线16设置", "曲线17设置", "曲线18设置", "曲线19设置", "曲线20设置", "曲线21设置", "曲线22设置", "曲线23设置", "曲线24设置", "曲线25设置", "曲线26设置", "曲线27设置", "曲线28设置", "曲线29设置", "曲线30设置", "曲线31设置", "曲线32设置", "曲线33设置", "曲线34设置", "曲线35设置", "曲线36设置", "曲线37设置", "曲线38设置", "曲线39设置", "曲线40设置", "曲线41设置", "曲线42设置", "曲线43设置", "曲线44设置", "曲线45设置", "曲线46设置", "曲线47设置", "曲线48设置", "曲线49设置", "曲线50设置", "曲线51设置", "曲线52设置", "曲线53设置", "曲线54设置", "曲线55设置", "曲线56设置", "曲线57设置", "曲线58设置", "曲线59设置", "曲线60设置", "曲线61设置", "曲线62设置", "曲线63设置", "曲线64设置", "ID值", "数据模式"] ("DataInitDef")
                    n785 = property on="表格" class="Tbl (严格)"() -> ("Selection Start"=w996:T1)  [unwired: 2 in, 2 out]
                    n786 = Unbundle By Name(w996) -> ("Row"=w994:i32)
                    n787 = property on="表格" class="Tbl (严格)"() -> ("Value"=w995:string[][])  [unwired: 2 in, 2 out]
                    n788 = Number To Decimal String(number=w994) -> (decimal integer string=w993:string)  [unwired: 1 in]
                    n789 = Index Array(array=w995, index (row)=w994, index (col)=0 ("禁用的索引 (列)")) -> (element=w992:string)
                    n790 = String Subset(string=w992, length (rest)=16 ("长度（剩余）")) -> (substring=w991:string)  [unwired: 1 in]
                    n791 = property on="曲线23设置" class="Str"("Val(Sgnl)"=w991) -> ()  [unwired: 2 in, 2 out]
                    n792 = invoke on="控件配置文件" class="Tbl (严格)" method="Set Cell Value"("X Index"=1 ("X索引"), "Y Index"=w986, "Value"=w993) -> ()  [unwired: 3 in, 6 out]
                    n793 = invoke on="控件配置文件" class="Tbl (严格)" method="Set Cell Value"("X Index"=0 ("X索引"), "Y Index"=w986, "Value"=w991) -> ()  [unwired: 3 in, 6 out]
                  }
                  frame "关联到曲线24" {
                    w997 = T9 53 items=["刷新间隔", "波特率", "布尔1设置项", "布尔2设置项", "布尔3设置项", "布尔4设置项", "布尔5设置项", "布尔6设置项", "布尔7设置项", "布尔8设置项", "显控1设置", "显控2设置", "显控3设置", "显控4设置", "显控5设置", "显控6设置", "显控7设置", "显控8设置", "显控9设置", "显控10设置", "显控11设置", "显控12设置", "设控1设置", "设控2设置", "设控3设置", "设控4设置", "设控5设置", "设控6设置", "设控7设置", "设控8设置", "曲线1设置", "曲线2设置", "曲线3设置", "曲线4设置", "曲线5设置", "曲线6设置", "曲线7设置", "曲线8设置", "曲线9设置", "曲线10设置", "曲线11设置", "曲线12设置", "曲线13设置", "曲线14设置", "曲线15设置", "曲线16设置", "曲线17设置", "曲线18设置", "曲线19设置", "曲线20设置", "曲线21设置", "曲线22设置", "曲线23设置", "曲线24设置", "曲线25设置", "曲线26设置", "曲线27设置", "曲线28设置", "曲线29设置", "曲线30设置", "曲线31设置", "曲线32设置", "曲线33设置", "曲线34设置", "曲线35设置", "曲线36设置", "曲线37设置", "曲线38设置", "曲线39设置", "曲线40设置", "曲线41设置", "曲线42设置", "曲线43设置", "曲线44设置", "曲线45设置", "曲线46设置", "曲线47设置", "曲线48设置", "曲线49设置", "曲线50设置", "曲线51设置", "曲线52设置", "曲线53设置", "曲线54设置", "曲线55设置", "曲线56设置", "曲线57设置", "曲线58设置", "曲线59设置", "曲线60设置", "曲线61设置", "曲线62设置", "曲线63设置", "曲线64设置", "ID值", "数据模式"] ("DataInitDef")
                    n794 = property on="表格" class="Tbl (严格)"() -> ("Selection Start"=w1007:T1)  [unwired: 2 in, 2 out]
                    n795 = Unbundle By Name(w1007) -> ("Row"=w1005:i32)
                    n796 = property on="表格" class="Tbl (严格)"() -> ("Value"=w1006:string[][])  [unwired: 2 in, 2 out]
                    n797 = Number To Decimal String(number=w1005) -> (decimal integer string=w1004:string)  [unwired: 1 in]
                    n798 = Index Array(array=w1006, index (row)=w1005, index (col)=0 ("禁用的索引 (列)")) -> (element=w1003:string)
                    n799 = String Subset(string=w1003, length (rest)=16 ("长度（剩余）")) -> (substring=w1002:string)  [unwired: 1 in]
                    n800 = property on="曲线24设置" class="Str"("Val(Sgnl)"=w1002) -> ()  [unwired: 2 in, 2 out]
                    n801 = invoke on="控件配置文件" class="Tbl (严格)" method="Set Cell Value"("X Index"=1 ("X索引"), "Y Index"=w997, "Value"=w1004) -> ()  [unwired: 3 in, 6 out]
                    n802 = invoke on="控件配置文件" class="Tbl (严格)" method="Set Cell Value"("X Index"=0 ("X索引"), "Y Index"=w997, "Value"=w1002) -> ()  [unwired: 3 in, 6 out]
                  }
                  frame "关联到曲线25" {
                    w1008 = T9 54 items=["刷新间隔", "波特率", "布尔1设置项", "布尔2设置项", "布尔3设置项", "布尔4设置项", "布尔5设置项", "布尔6设置项", "布尔7设置项", "布尔8设置项", "显控1设置", "显控2设置", "显控3设置", "显控4设置", "显控5设置", "显控6设置", "显控7设置", "显控8设置", "显控9设置", "显控10设置", "显控11设置", "显控12设置", "设控1设置", "设控2设置", "设控3设置", "设控4设置", "设控5设置", "设控6设置", "设控7设置", "设控8设置", "曲线1设置", "曲线2设置", "曲线3设置", "曲线4设置", "曲线5设置", "曲线6设置", "曲线7设置", "曲线8设置", "曲线9设置", "曲线10设置", "曲线11设置", "曲线12设置", "曲线13设置", "曲线14设置", "曲线15设置", "曲线16设置", "曲线17设置", "曲线18设置", "曲线19设置", "曲线20设置", "曲线21设置", "曲线22设置", "曲线23设置", "曲线24设置", "曲线25设置", "曲线26设置", "曲线27设置", "曲线28设置", "曲线29设置", "曲线30设置", "曲线31设置", "曲线32设置", "曲线33设置", "曲线34设置", "曲线35设置", "曲线36设置", "曲线37设置", "曲线38设置", "曲线39设置", "曲线40设置", "曲线41设置", "曲线42设置", "曲线43设置", "曲线44设置", "曲线45设置", "曲线46设置", "曲线47设置", "曲线48设置", "曲线49设置", "曲线50设置", "曲线51设置", "曲线52设置", "曲线53设置", "曲线54设置", "曲线55设置", "曲线56设置", "曲线57设置", "曲线58设置", "曲线59设置", "曲线60设置", "曲线61设置", "曲线62设置", "曲线63设置", "曲线64设置", "ID值", "数据模式"] ("DataInitDef")
                    n803 = property on="表格" class="Tbl (严格)"() -> ("Selection Start"=w1018:T1)  [unwired: 2 in, 2 out]
                    n804 = Unbundle By Name(w1018) -> ("Row"=w1016:i32)
                    n805 = property on="表格" class="Tbl (严格)"() -> ("Value"=w1017:string[][])  [unwired: 2 in, 2 out]
                    n806 = Number To Decimal String(number=w1016) -> (decimal integer string=w1015:string)  [unwired: 1 in]
                    n807 = Index Array(array=w1017, index (row)=w1016, index (col)=0 ("禁用的索引 (列)")) -> (element=w1014:string)
                    n808 = String Subset(string=w1014, length (rest)=16 ("长度（剩余）")) -> (substring=w1013:string)  [unwired: 1 in]
                    n809 = property on="曲线25设置" class="Str"("Val(Sgnl)"=w1013) -> ()  [unwired: 2 in, 2 out]
                    n810 = invoke on="控件配置文件" class="Tbl (严格)" method="Set Cell Value"("X Index"=1 ("X索引"), "Y Index"=w1008, "Value"=w1015) -> ()  [unwired: 3 in, 6 out]
                    n811 = invoke on="控件配置文件" class="Tbl (严格)" method="Set Cell Value"("X Index"=0 ("X索引"), "Y Index"=w1008, "Value"=w1013) -> ()  [unwired: 3 in, 6 out]
                  }
                  frame "关联到曲线26" {
                    w1019 = T9 55 items=["刷新间隔", "波特率", "布尔1设置项", "布尔2设置项", "布尔3设置项", "布尔4设置项", "布尔5设置项", "布尔6设置项", "布尔7设置项", "布尔8设置项", "显控1设置", "显控2设置", "显控3设置", "显控4设置", "显控5设置", "显控6设置", "显控7设置", "显控8设置", "显控9设置", "显控10设置", "显控11设置", "显控12设置", "设控1设置", "设控2设置", "设控3设置", "设控4设置", "设控5设置", "设控6设置", "设控7设置", "设控8设置", "曲线1设置", "曲线2设置", "曲线3设置", "曲线4设置", "曲线5设置", "曲线6设置", "曲线7设置", "曲线8设置", "曲线9设置", "曲线10设置", "曲线11设置", "曲线12设置", "曲线13设置", "曲线14设置", "曲线15设置", "曲线16设置", "曲线17设置", "曲线18设置", "曲线19设置", "曲线20设置", "曲线21设置", "曲线22设置", "曲线23设置", "曲线24设置", "曲线25设置", "曲线26设置", "曲线27设置", "曲线28设置", "曲线29设置", "曲线30设置", "曲线31设置", "曲线32设置", "曲线33设置", "曲线34设置", "曲线35设置", "曲线36设置", "曲线37设置", "曲线38设置", "曲线39设置", "曲线40设置", "曲线41设置", "曲线42设置", "曲线43设置", "曲线44设置", "曲线45设置", "曲线46设置", "曲线47设置", "曲线48设置", "曲线49设置", "曲线50设置", "曲线51设置", "曲线52设置", "曲线53设置", "曲线54设置", "曲线55设置", "曲线56设置", "曲线57设置", "曲线58设置", "曲线59设置", "曲线60设置", "曲线61设置", "曲线62设置", "曲线63设置", "曲线64设置", "ID值", "数据模式"] ("DataInitDef")
                    n812 = property on="表格" class="Tbl (严格)"() -> ("Selection Start"=w1029:T1)  [unwired: 2 in, 2 out]
                    n813 = Unbundle By Name(w1029) -> ("Row"=w1027:i32)
                    n814 = property on="表格" class="Tbl (严格)"() -> ("Value"=w1028:string[][])  [unwired: 2 in, 2 out]
                    n815 = Number To Decimal String(number=w1027) -> (decimal integer string=w1026:string)  [unwired: 1 in]
                    n816 = Index Array(array=w1028, index (row)=w1027, index (col)=0 ("禁用的索引 (列)")) -> (element=w1025:string)
                    n817 = String Subset(string=w1025, length (rest)=16 ("长度（剩余）")) -> (substring=w1024:string)  [unwired: 1 in]
                    n818 = property on="曲线26设置" class="Str"("Val(Sgnl)"=w1024) -> ()  [unwired: 2 in, 2 out]
                    n819 = invoke on="控件配置文件" class="Tbl (严格)" method="Set Cell Value"("X Index"=1 ("X索引"), "Y Index"=w1019, "Value"=w1026) -> ()  [unwired: 3 in, 6 out]
                    n820 = invoke on="控件配置文件" class="Tbl (严格)" method="Set Cell Value"("X Index"=0 ("X索引"), "Y Index"=w1019, "Value"=w1024) -> ()  [unwired: 3 in, 6 out]
                  }
                  frame "关联到曲线27" {
                    w1030 = T9 56 items=["刷新间隔", "波特率", "布尔1设置项", "布尔2设置项", "布尔3设置项", "布尔4设置项", "布尔5设置项", "布尔6设置项", "布尔7设置项", "布尔8设置项", "显控1设置", "显控2设置", "显控3设置", "显控4设置", "显控5设置", "显控6设置", "显控7设置", "显控8设置", "显控9设置", "显控10设置", "显控11设置", "显控12设置", "设控1设置", "设控2设置", "设控3设置", "设控4设置", "设控5设置", "设控6设置", "设控7设置", "设控8设置", "曲线1设置", "曲线2设置", "曲线3设置", "曲线4设置", "曲线5设置", "曲线6设置", "曲线7设置", "曲线8设置", "曲线9设置", "曲线10设置", "曲线11设置", "曲线12设置", "曲线13设置", "曲线14设置", "曲线15设置", "曲线16设置", "曲线17设置", "曲线18设置", "曲线19设置", "曲线20设置", "曲线21设置", "曲线22设置", "曲线23设置", "曲线24设置", "曲线25设置", "曲线26设置", "曲线27设置", "曲线28设置", "曲线29设置", "曲线30设置", "曲线31设置", "曲线32设置", "曲线33设置", "曲线34设置", "曲线35设置", "曲线36设置", "曲线37设置", "曲线38设置", "曲线39设置", "曲线40设置", "曲线41设置", "曲线42设置", "曲线43设置", "曲线44设置", "曲线45设置", "曲线46设置", "曲线47设置", "曲线48设置", "曲线49设置", "曲线50设置", "曲线51设置", "曲线52设置", "曲线53设置", "曲线54设置", "曲线55设置", "曲线56设置", "曲线57设置", "曲线58设置", "曲线59设置", "曲线60设置", "曲线61设置", "曲线62设置", "曲线63设置", "曲线64设置", "ID值", "数据模式"] ("DataInitDef")
                    n821 = property on="表格" class="Tbl (严格)"() -> ("Selection Start"=w1040:T1)  [unwired: 2 in, 2 out]
                    n822 = Unbundle By Name(w1040) -> ("Row"=w1038:i32)
                    n823 = property on="表格" class="Tbl (严格)"() -> ("Value"=w1039:string[][])  [unwired: 2 in, 2 out]
                    n824 = Number To Decimal String(number=w1038) -> (decimal integer string=w1037:string)  [unwired: 1 in]
                    n825 = Index Array(array=w1039, index (row)=w1038, index (col)=0 ("禁用的索引 (列)")) -> (element=w1036:string)
                    n826 = String Subset(string=w1036, length (rest)=16 ("长度（剩余）")) -> (substring=w1035:string)  [unwired: 1 in]
                    n827 = property on="曲线27设置" class="Str"("Val(Sgnl)"=w1035) -> ()  [unwired: 2 in, 2 out]
                    n828 = invoke on="控件配置文件" class="Tbl (严格)" method="Set Cell Value"("X Index"=1 ("X索引"), "Y Index"=w1030, "Value"=w1037) -> ()  [unwired: 3 in, 6 out]
                    n829 = invoke on="控件配置文件" class="Tbl (严格)" method="Set Cell Value"("X Index"=0 ("X索引"), "Y Index"=w1030, "Value"=w1035) -> ()  [unwired: 3 in, 6 out]
                  }
                  frame "关联到曲线28" {
                    w1041 = T9 57 items=["刷新间隔", "波特率", "布尔1设置项", "布尔2设置项", "布尔3设置项", "布尔4设置项", "布尔5设置项", "布尔6设置项", "布尔7设置项", "布尔8设置项", "显控1设置", "显控2设置", "显控3设置", "显控4设置", "显控5设置", "显控6设置", "显控7设置", "显控8设置", "显控9设置", "显控10设置", "显控11设置", "显控12设置", "设控1设置", "设控2设置", "设控3设置", "设控4设置", "设控5设置", "设控6设置", "设控7设置", "设控8设置", "曲线1设置", "曲线2设置", "曲线3设置", "曲线4设置", "曲线5设置", "曲线6设置", "曲线7设置", "曲线8设置", "曲线9设置", "曲线10设置", "曲线11设置", "曲线12设置", "曲线13设置", "曲线14设置", "曲线15设置", "曲线16设置", "曲线17设置", "曲线18设置", "曲线19设置", "曲线20设置", "曲线21设置", "曲线22设置", "曲线23设置", "曲线24设置", "曲线25设置", "曲线26设置", "曲线27设置", "曲线28设置", "曲线29设置", "曲线30设置", "曲线31设置", "曲线32设置", "曲线33设置", "曲线34设置", "曲线35设置", "曲线36设置", "曲线37设置", "曲线38设置", "曲线39设置", "曲线40设置", "曲线41设置", "曲线42设置", "曲线43设置", "曲线44设置", "曲线45设置", "曲线46设置", "曲线47设置", "曲线48设置", "曲线49设置", "曲线50设置", "曲线51设置", "曲线52设置", "曲线53设置", "曲线54设置", "曲线55设置", "曲线56设置", "曲线57设置", "曲线58设置", "曲线59设置", "曲线60设置", "曲线61设置", "曲线62设置", "曲线63设置", "曲线64设置", "ID值", "数据模式"] ("DataInitDef")
                    n830 = property on="表格" class="Tbl (严格)"() -> ("Selection Start"=w1051:T1)  [unwired: 2 in, 2 out]
                    n831 = Unbundle By Name(w1051) -> ("Row"=w1049:i32)
                    n832 = property on="表格" class="Tbl (严格)"() -> ("Value"=w1050:string[][])  [unwired: 2 in, 2 out]
                    n833 = Number To Decimal String(number=w1049) -> (decimal integer string=w1048:string)  [unwired: 1 in]
                    n834 = Index Array(array=w1050, index (row)=w1049, index (col)=0 ("禁用的索引 (列)")) -> (element=w1047:string)
                    n835 = String Subset(string=w1047, length (rest)=16 ("长度（剩余）")) -> (substring=w1046:string)  [unwired: 1 in]
                    n836 = property on="曲线28设置" class="Str"("Val(Sgnl)"=w1046) -> ()  [unwired: 2 in, 2 out]
                    n837 = invoke on="控件配置文件" class="Tbl (严格)" method="Set Cell Value"("X Index"=1 ("X索引"), "Y Index"=w1041, "Value"=w1048) -> ()  [unwired: 3 in, 6 out]
